vi "Temperature Monitoring.vi"() -> ()   [LabVIEW 2023]
doc: "Temperature Monitoring.vi demonstrates a temperature monitoring application. This VI reads a simulated temperature and alarms if it is outside a given range."
uses:
  controls/Temp Monitor UI Data.ctl
  <vilib>/Utility/error.llb/Error Cluster From Error Code.vi
  <vilib>/ErrorRing/Error Ring.xnode
  support/User Event - Stop/Temp Monitor User Event - Stop.lvlib
  support/Message Queue/Temp Monitor Message Queue.lvlib
panel:
  out "Alarm":string
  in  "Low Limit":dbl(slide)=75.0 scale=70.0..90.0 scale format="%0.0f"
  in  "High Limit":dbl(slide)=85.0 scale=70.0..90.0 scale format="%0.0f"
  out "Temperature (F)":dbl
  out "Temperature History":T1(graph)
  in  "Start":bool
  in  "Stop":bool
  out "Status":string
  in  "Exit":bool
  # "Overview: Demonstrates a temperature monitoring system built from the Continuous Measurement and Logging sample project.\nInstructions:\n1. Run the VI.\n2. Click the Start button to start monitoring temperature data.\n3. Click the Stop button to stop monitoring temperature data.\n4. Click Exit to stop the VI."
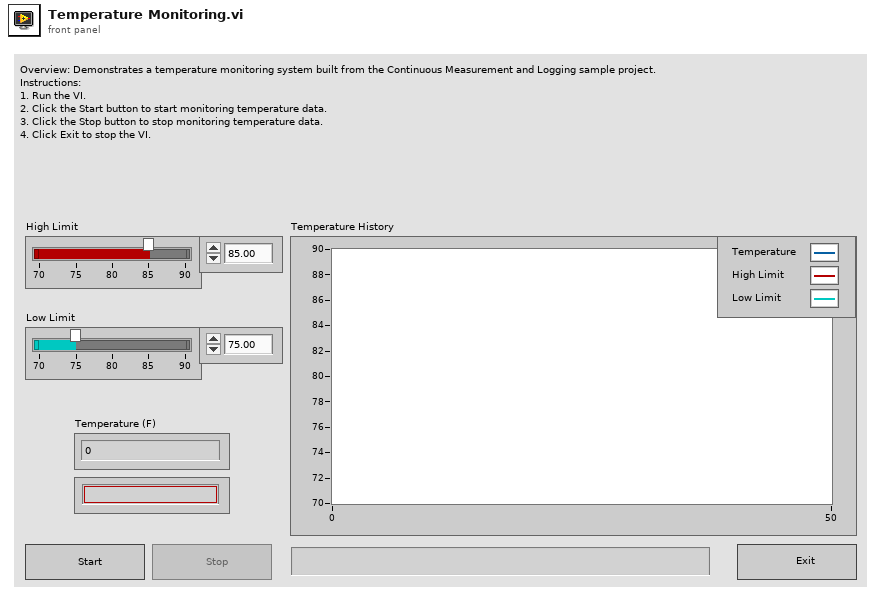
[diagram p1: front panel]
types:
  T1 = cluster{"temperature":dbl, "High Limit":dbl, "Low Limit":dbl}
  T2 = typedef "Temp Monitor UI Data.ctl" = cluster{"Start Ref":refnum<vi>, "Stop Ref":refnum<vi>, "Exit Ref":refnum<vi>}
  T3 = typedef "Temp Monitor Message Queue.lvlib/All Message Queues.ctl" = cluster{"UI":refnum<queue>, "Acquisition":refnum<queue>}
  T4 = typedef "Simulated Data.ctl" = cluster{"temperature":dbl, "High Limit":dbl, "Low Limit":dbl}
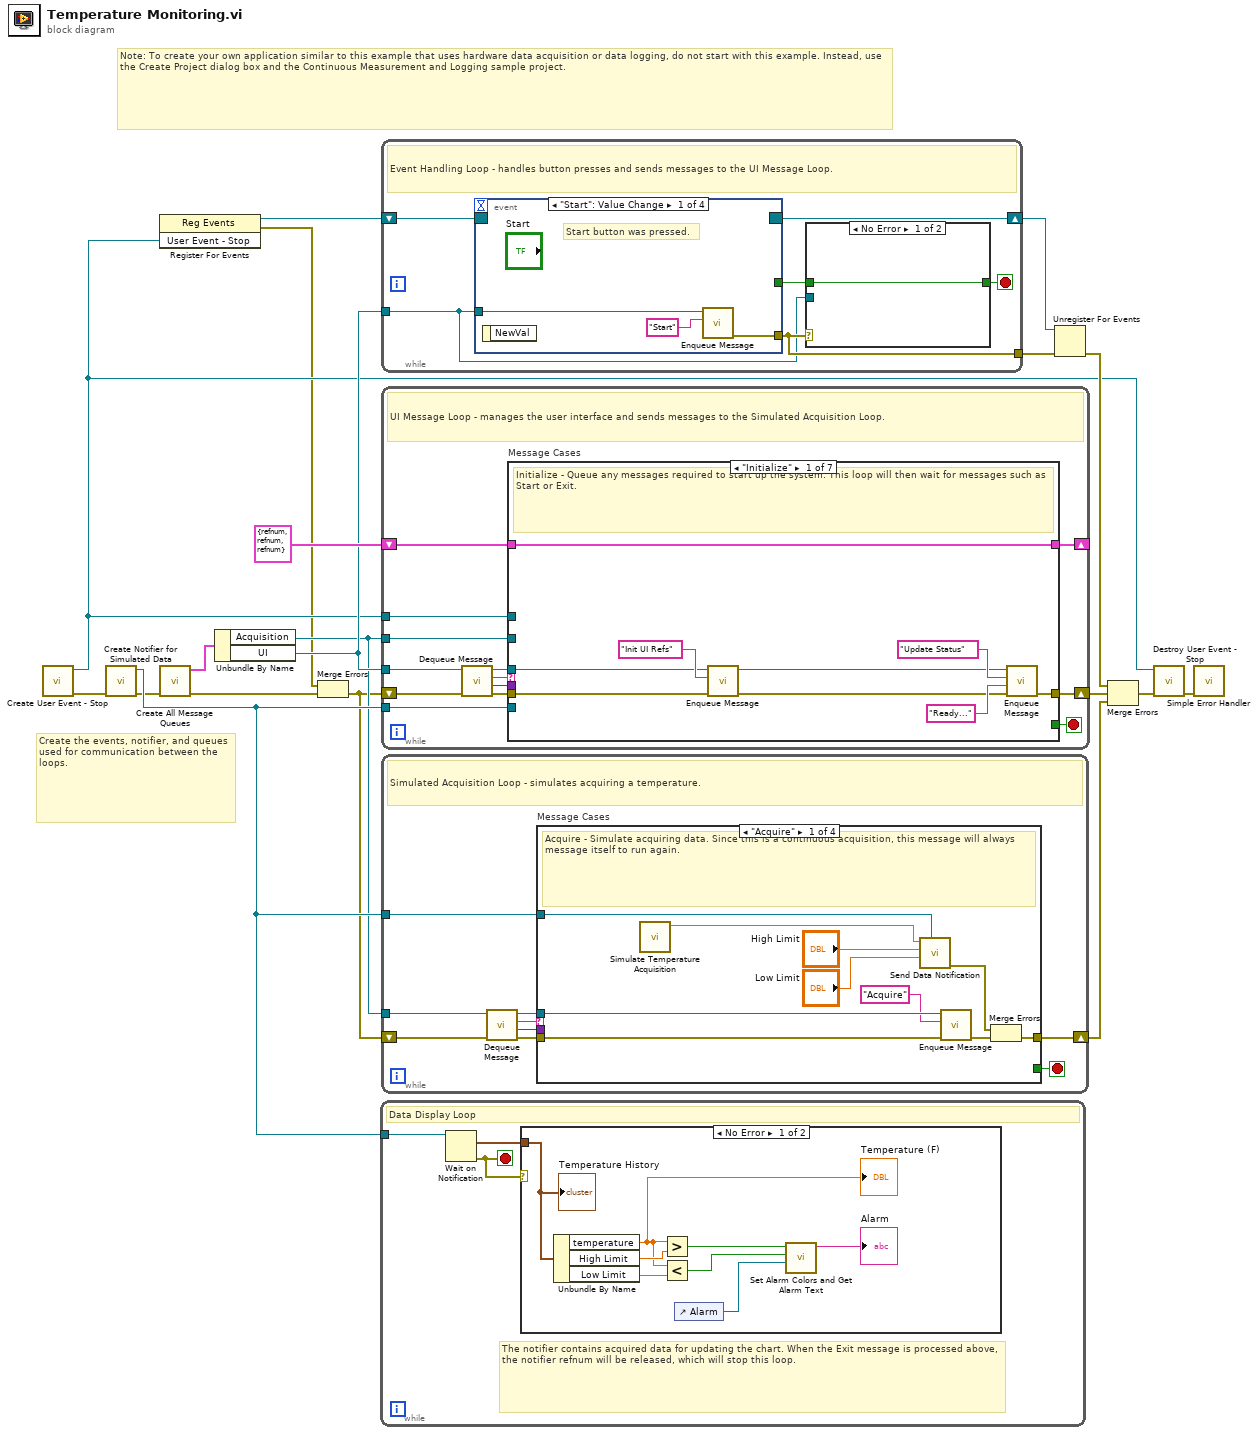
[diagram p0: block diagram]
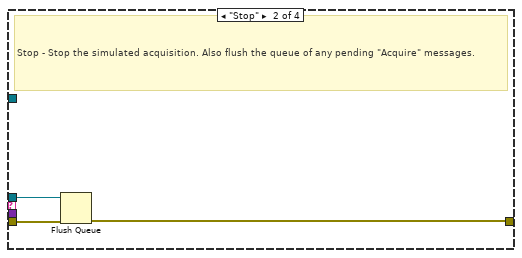
[diagram p2: hidden frame]
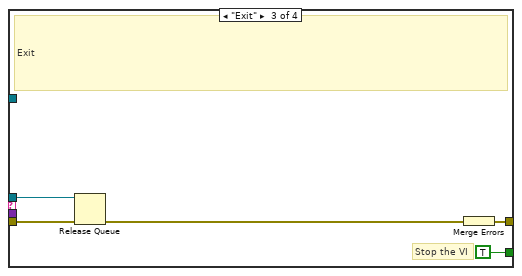
[diagram p3: hidden frame]
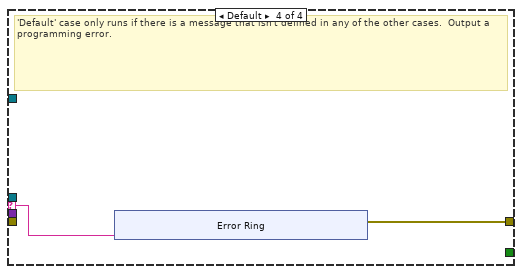
[diagram p4: hidden frame]
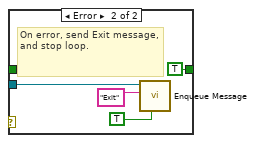
[diagram p6: hidden frame]
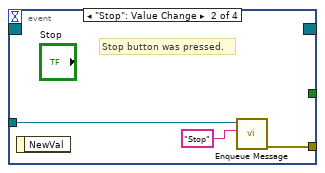
[diagram p7: hidden frame]
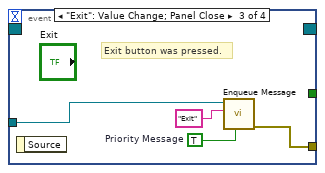
[diagram p8: hidden frame]
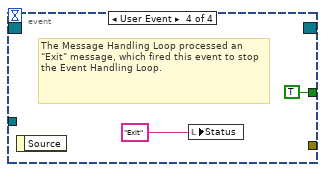
[diagram p9: hidden frame]
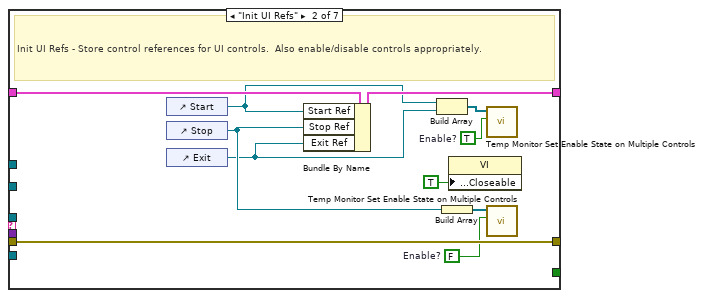
[diagram p10: hidden frame]
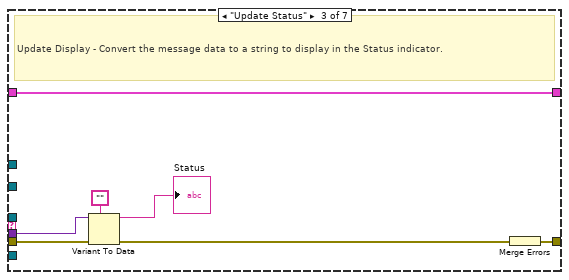
[diagram p11: hidden frame]
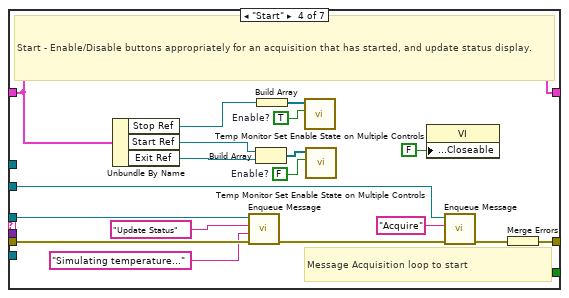
[diagram p12: hidden frame]
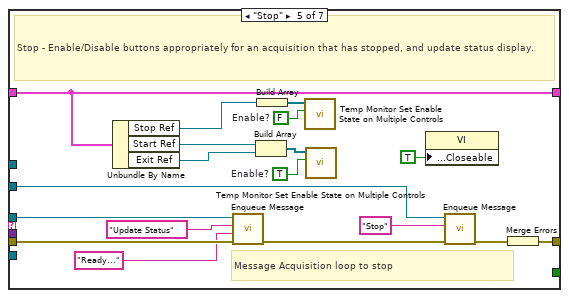
[diagram p13: hidden frame]
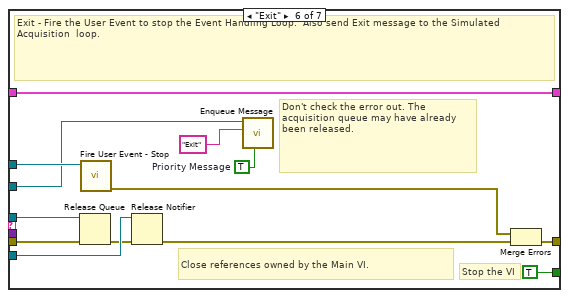
[diagram p14: hidden frame]
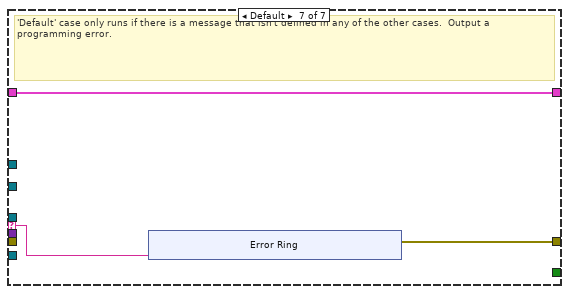
[diagram p15: hidden frame]
diagram:
  # "Note: To create your own application similar to this example that uses hardware data acquisition or data logging, do not start with this example. Instead, use the Create Project dialog box and the Continuous Measurement and Logging sample project."
  # "Create the events, notifier, and queues used for communication between the loops."
  n1 = call "Create User Event - Stop.vi"() -> ("error out"=w7:errorcluster, "User Event - Stop"=w3:refnum<user-event>)  [unwired: 10 in]
  n2 = call "Create Notifier for Simulated Data.vi"("error in (no error)"=w7) -> ("error out"=w6:errorcluster, "Notifier out"=w10:refnum<notifier>)  [unwired: 9 in]
  n3 = register-events(w3) -> (reference out=w4:refnum<event-registration>, error out=w1:errorcluster)  [unwired: 2 in]
  n4 = call "Create All Message Queues.vi"("error in (no error)"=w6) -> ("error out"=w5:errorcluster, "Message Queues out"=w16:T3)  [unwired: 9 in]
  n5 = Unbundle By Name(w16) -> ("Acquisition"=w8:refnum<queue>, "UI"=w9:refnum<queue>)
  n6 = Merge Errors(w1, w5) -> (w2:errorcluster)
  n7 = while "Data Display Loop" {
    tunnel: w10 -> [w22]
    stop <- w20 stop-if-true
    # "The notifier contains acquired data for updating the chart. When the Exit message is processed above, the notifier refnum will be released, which will stop this loop."
    # "Data Display Loop"
    n8 = Wait on Notification(notifier=w22) -> (notification=w21:T4, error out=w20:errorcluster)  [unwired: 3 in, 2 out]
    n9 = case shown="No Error" w20 {
      tunnel: w21 -> [w30 _]
      frame No Error {
        n10 = Unbundle By Name(w30) -> ("temperature"=w27:dbl, "High Limit"=w29:dbl, "Low Limit"=w28:dbl)
        "Temperature (F)" <- w27
        n11 = Greater?(x=w27, y=w29) -> (0:w26:bool)
        n12 = Less?(x=w27, y=w28) -> (x < y?=w25:bool)
        n13 = control-ref of="Alarm"() -> (w24:refnum<vi>)
        n14 = call "Set Alarm Colors and Get Alarm Text.vi"("Alarm reference"=w24, "Under Low Limit"=w25, "Over High Limit"=w26) -> ("Alarm String"=→"Alarm":string)  [unwired: 8 in]
        "Temperature History" <- w30
      }
      frame Error {
      }
    }
  }
  n15 = while {
    tunnel: w9 -> [w32]
    tunnel: [w34] -> w18
    shift-right: [w31] -> w14
    shift-left: w4 -> [w33]
    stop <- w35 stop-if-true
    # "Event Handling Loop - handles button presses and sends messages to the UI Message Loop."
    n16 = event shown="[0] \"Start\": Value Change" {
      selector: w33 -> [_ _ _ _]
      dyn-events: [_ _ _ _] -> w31
      timeout: _ -> [_ _ _ _]
      tunnel: [_ _ _ TRUE ("Discard?")] -> w36
      tunnel: w32 -> [w42 w46 w48 _]
      tunnel: [w44 w45 w51 _] -> w34
      event "Start": Value Change {
        # "Start button was pressed."
        n17 = event-data() -> ()  [unwired: 1 in, 1 out]
        n18 = call "Enqueue Message.vi"("Message"="Start", "Message Queue"=w42) -> ("error out"=w44:errorcluster)  [unwired: 8 in, 1 out]
      }
      event "Stop": Value Change {
        # "Stop button was pressed."
        n19 = event-data() -> ()  [unwired: 1 in, 1 out]
        n20 = call "Enqueue Message.vi"("Message"="Stop", "Message Queue"=w46) -> ("error out"=w45:errorcluster)  [unwired: 8 in, 1 out]
      }
      event "Exit": Value Change; Panel Close {
        w49 = TRUE  # Priority Message
        # "Exit button was pressed."
        n21 = event-data() -> ()  [unwired: 1 in, 1 out]
        n22 = call "Enqueue Message.vi"("Priority Message? (F)"=w49, "Message"="Exit", "Message Queue"=w48) -> ("error out"=w51:errorcluster)  [unwired: 7 in, 1 out]
      }
      event User Event {
        # "The Message Handling Loop processed an \"Exit\" message, which fired this event to stop the Event Handling Loop."
        n23 = event-data() -> ()  [unwired: 1 in, 1 out]
        n24 = local write "Status"("Exit" ("Exit String")) -> ()
      }
    }
    n25 = case shown="No Error" w34 {
      tunnel: [w37 TRUE ("Discard?")] -> w35
      tunnel: w36 -> [w37 _]
      tunnel: w32 -> [_ w38]
      frame No Error {
      }
      frame Error {
        # "On error, send Exit message, and stop loop."
        n26 = call "Enqueue Message.vi"("Priority Message? (F)"=TRUE ("Discard?"), "Message"="Exit", "Message Queue"=w38) -> ()  [unwired: 7 in, 2 out]
      }
    }
  }
  n27 = while {
    tunnel: w9 -> [w58]
    tunnel: w3 -> [w64]
    shift-right: [w65] -> w19
    shift-left: w2 -> [w63]
    shift-right: [w56] -> _
    shift-left: T2 {"Start Ref"=refnum, "Stop Ref"=refnum, "Exit Ref"=refnum} ("Measurement UI Controls") -> [w57]
    tunnel: w8 -> [w55]
    tunnel: w10 -> [w54]
    stop <- w66 stop-if-true
    # "UI Message Loop - manages the user interface and sends messages to the Simulated Acquisition Loop."
    n28 = call "Dequeue Message.vi"("error in (no error)"=w63, "Message Queue"=w58) -> ("error out"=w62:errorcluster, "Message Data"=w60:variant, "Message"=w61:string, "dup Message Queue"=w59:refnum<queue>)  [unwired: 6 in]
    n29 = case "Message Cases" shown="\"Initialize\"" w61 {
      selector: w61 -> [_ _ _ _ _ _ w143]
      tunnel: w59 -> [w70 _ _ w110 w128 w134 _]
      tunnel: w62 -> [w69 w86 w92 w109 w127 w140 _]
      tunnel: [w75 w86 w93 w111 w129 w141 w144] -> w65
      tunnel: [_ _ _ _ _ TRUE _] -> w66
      tunnel: w60 -> [_ _ w91 _ _ _ _]
      tunnel: w64 -> [_ _ _ _ _ w139 _]
      tunnel: w57 -> [w72 w85 w87 w94 w112 w136 w145]
      tunnel: [w72 w84 w87 w94 w112 w136 w145] -> w56
      tunnel: w55 -> [_ _ _ w98 w116 w135 _]
      tunnel: w54 -> [_ _ _ _ _ w133 _]
      frame "Initialize" {
        # "Initialize - Queue any messages required to start up the system. This loop will then wait for messages such as Start or Exit."
        n30 = call "Enqueue Message.vi"("error in (no error)"=w69, "Message"="Init UI Refs", "Message Queue"=w70) -> ("error out"=w67:errorcluster, "dup Message Queue"=w68:refnum<queue>)  [unwired: 7 in]
        n31 = call "Enqueue Message.vi"("error in (no error)"=w67, "Message Data"="Ready..." ("Ready..."), "Message"="Update Status", "Message Queue"=w68) -> ("error out"=w75:errorcluster)  [unwired: 6 in, 1 out]
      }
      frame "Init UI Refs" {
        w80 = FALSE  # Enable?
        w83 = TRUE  # Enable?
        # "Init UI Refs - Store control references for UI controls.  Also enable/disable controls appropriately."
        n32 = control-ref of="Start"() -> (w76:refnum<vi>)
        n33 = control-ref of="Stop"() -> (w79:refnum<vi>)
        n34 = control-ref of="Exit"() -> (w77:refnum<vi>)
        n35 = Bundle By Name(cluster=w85, "Start Ref"=w76, "Stop Ref"=w79, "Exit Ref"=w77) -> (w84:T2)
        n36 = Build Array(w76, w77) -> (w82:refnum<vi>[])
        n37 = Build Array(w79) -> (w81:refnum<vi>[])
        n38 = property class="VI"("Front Panel.Closeable"=TRUE) -> ()  [unwired: 2 in, 2 out]
        n39 = call "Temp Monitor Set Enable State on Multiple Controls.vi"("Enable?"=w83, "Controls"=w82) -> ()  [unwired: 10 in]
        n40 = call "Temp Monitor Set Enable State on Multiple Controls.vi"("Enable?"=w80, "Controls"=w81) -> ()  [unwired: 10 in]
      }
      frame "Update Status" {
        # "Update Display - Convert the message data to a string to display in the Status indicator."
        n41 = Variant To Data(error in=w92, type="", Variant=w91) -> (data=→"Status":string, error out=w89:errorcluster)
        n42 = Merge Errors(w89) -> (w93:errorcluster)
      }
      frame "Start" {
        w103 = TRUE  # Enable?
        w106 = FALSE  # Enable?
        # "Message Acquisition loop to start"
        # "Start - Enable/Disable buttons appropriately for an acquisition that has started, and update status display."
        n43 = Unbundle By Name(w94) -> ("Stop Ref"=w102:refnum<vi>, "Start Ref"=w101:refnum<vi>, "Exit Ref"=w100:refnum<vi>)
        n44 = call "Enqueue Message.vi"("error in (no error)"=w109, "Message Data"="Simulating temperature..." ("Acquiring and Logging..."), "Message"="Update Status", "Message Queue"=w110) -> ("error out"=w95:errorcluster)  [unwired: 6 in, 1 out]
        n45 = Build Array(w101, w100) -> (w105:refnum<vi>[])
        n46 = Build Array(w102) -> (w104:refnum<vi>[])
        n47 = call "Temp Monitor Set Enable State on Multiple Controls.vi"("Enable?"=w103, "Controls"=w104) -> ()  [unwired: 10 in]
        n48 = call "Temp Monitor Set Enable State on Multiple Controls.vi"("Enable?"=w106, "Controls"=w105) -> ()  [unwired: 10 in]
        n49 = property class="VI"("Front Panel.Closeable"=FALSE) -> ()  [unwired: 2 in, 2 out]
        n50 = call "Enqueue Message.vi"("error in (no error)"=w95, "Message"="Acquire", "Message Queue"=w98) -> ("error out"=w99:errorcluster)  [unwired: 7 in, 1 out]
        n51 = Merge Errors(w99) -> (w111:errorcluster)
      }
      frame "Stop" {
        w121 = FALSE  # Enable?
        w124 = TRUE  # Enable?
        # "Message Acquisition loop to stop"
        # "Stop - Enable/Disable buttons appropriately for an acquisition that has stopped, and update status display."
        n52 = Unbundle By Name(w112) -> ("Stop Ref"=w120:refnum<vi>, "Start Ref"=w119:refnum<vi>, "Exit Ref"=w118:refnum<vi>)
        n53 = call "Enqueue Message.vi"("error in (no error)"=w127, "Message Data"="Ready..." ("Ready..."), "Message"="Update Status", "Message Queue"=w128) -> ("error out"=w113:errorcluster)  [unwired: 6 in, 1 out]
        n54 = Build Array(w119, w118) -> (w123:refnum<vi>[])
        n55 = Build Array(w120) -> (w122:refnum<vi>[])
        n56 = call "Temp Monitor Set Enable State on Multiple Controls.vi"("Enable?"=w121, "Controls"=w122) -> ()  [unwired: 10 in]
        n57 = call "Temp Monitor Set Enable State on Multiple Controls.vi"("Enable?"=w124, "Controls"=w123) -> ()  [unwired: 10 in]
        n58 = property class="VI"("Front Panel.Closeable"=TRUE) -> ()  [unwired: 2 in, 2 out]
        n59 = call "Enqueue Message.vi"("error in (no error)"=w113, "Message"="Stop", "Message Queue"=w116) -> ("error out"=w117:errorcluster)  [unwired: 7 in, 1 out]
        n60 = Merge Errors(w117) -> (w129:errorcluster)
      }
      frame "Exit" {
        w130 = TRUE  # Priority Message
        # "Don't check the error out. The acquisition queue may have already been released."
        # "Close references owned by the Main VI."
        # "Stop the VI"
        # "Exit - Fire the User Event to stop the Event Handling Loop.  Also send Exit message to the Simulated Acquisition  loop."
        n61 = Release Queue(queue=w134, error in (no error)=w140) -> (error out=w132:errorcluster)  [unwired: 1 in, 2 out]
        n62 = call "Fire User Event - Stop.vi"("User Event - Stop"=w139) -> ("error out"=w138:errorcluster)  [unwired: 10 in]
        n63 = Release Notifier(notifier=w133, error in (no error)=w132) -> (error out=w131:errorcluster)  [unwired: 1 in, 2 out]
        n64 = call "Enqueue Message.vi"("Priority Message? (F)"=w130, "Message"="Exit", "Message Queue"=w135) -> ()  [unwired: 7 in, 2 out]
        n65 = Merge Errors(w138, w131) -> (w141:errorcluster)
      }
      frame Default {
        # "'Default' case only runs if there is a message that isn't defined in any of the other cases.  Output a programming error."
        n66 = xnode "Error Ring"("parameter 0"=w143) -> ("error out"=w144:errorcluster)
      }
    }
  }
  n67 = while {
    tunnel: w8 -> [w155]
    shift-right: [w160] -> w11
    shift-left: w2 -> [w159]
    tunnel: w10 -> [w154]
    stop <- w161 stop-if-true
    # "Simulated Acquisition Loop - simulates acquiring a temperature."
    n68 = call "Dequeue Message.vi"("error in (no error)"=w159, "Message Queue"=w155) -> ("error out"=w158:errorcluster, "Message Data"=w156:variant, "Message"=w157:string, "dup Message Queue"=w153:refnum<queue>)  [unwired: 6 in]
    n69 = case "Message Cases" shown="\"Acquire\"" w157 {
      selector: w157 -> [_ _ _ w180]
      tunnel: w153 -> [w169 w174 w177 _]
      tunnel: w158 -> [w168 w173 w176 _]
      tunnel: [w171 w172 w178 w181] -> w160
      tunnel: [_ _ TRUE _] -> w161
      tunnel: w156 -> [_ _ _ _]
      tunnel: w154 -> [w162 _ _ _]
      frame "Acquire" {
        # "Acquire - Simulate acquiring data. Since this is a continuous acquisition, this message will always message itself to run again."
        n70 = call "Simulate Temperature Acquisition.vi"() -> ("temperature"=w165:dbl)  [unwired: 11 in]
        n71 = call "Send Data Notification.vi"("Notifier in"=w162, "Low Limit"="Low Limit", "High Limit"="High Limit", "temperature"=w165) -> ("error out"=w166:errorcluster)  [unwired: 7 in]
        n72 = call "Enqueue Message.vi"("error in (no error)"=w168, "Message"="Acquire", "Message Queue"=w169) -> ("error out"=w170:errorcluster)  [unwired: 7 in, 1 out]
        n73 = Merge Errors(w166, w170) -> (w171:errorcluster)
      }
      frame "Stop" {
        # "Stop - Stop the simulated acquisition. Also flush the queue of any pending \"Acquire\" messages."
        n74 = Flush Queue(queue=w174, error in (no error)=w173) -> (error out=w172:errorcluster)  [unwired: 2 out]
      }
      frame "Exit" {
        # "Stop the VI"
        # "Exit"
        n75 = Release Queue(queue=w177, error in (no error)=w176) -> (error out=w175:errorcluster)  [unwired: 1 in, 2 out]
        n76 = Merge Errors(w175) -> (w178:errorcluster)
      }
      frame Default {
        # "'Default' case only runs if there is a message that isn't defined in any of the other cases.  Output a programming error."
        n77 = xnode "Error Ring"("parameter 0"=w180) -> ("error out"=w181:errorcluster)
      }
    }
  }
  n78 = Unregister For Events(event registration refnum=w14, error in=w18) -> (error out=w15:errorcluster)
  n79 = Merge Errors(w15, w19, w11) -> (w17:errorcluster)
  n80 = call "Destroy User Event - Stop.vi"("error in (no error)"=w17, "User Event - Stop"=w3) -> ("error out"=w12:errorcluster)  [unwired: 9 in]
  n81 = call <vilib>:"Simple Error Handler.vi"("error in (no error)"=w12) -> ()  [unwired: 4 in, 5 out]
